vi "功能计算_何 截取位移.vi"(0 "位移数组":dbl[](array[numeric]), 2 "拉压力数组":dbl[](array[numeric])) -> (14 "峰值扭矩":dbl format="%#.2f", 16 "最小扭矩":dbl, 17 "平均扭矩":dbl format="%#.2f", 19 "扭差":dbl format="%#.2f")   [LabVIEW 2013]
panel:
  in  "截取百分比":dbl
  in  "半行程":dbl
  out "第一个子数组":dbl[](array[numeric])
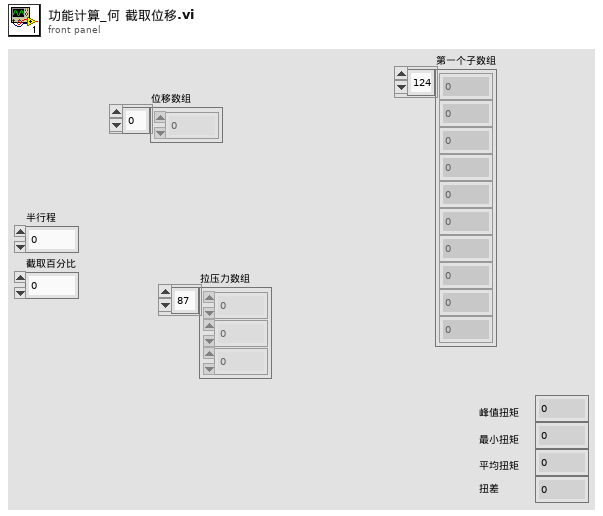
[diagram p1: front panel]
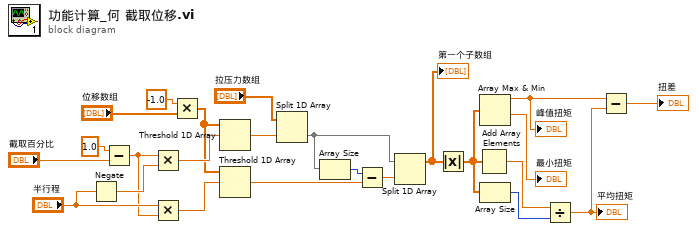
[diagram p0: block diagram]
diagram:
  n1 = Negate(x="半行程") -> (-x=w4:dbl)
  n2 = Subtract(x=1.0, y="截取百分比") -> (x-y=w3:dbl)
  n3 = Multiply(x=w3, y=w4) -> (x*y=w8:dbl)
  n4 = Multiply(x="半行程", y=w3) -> (x*y=w5:dbl)
  n5 = Multiply(x=-1.0, y="位移数组") -> (x*y=w7:dbl[])
  n6 = Threshold 1D Array(2:w8, 3:w7) -> (0:w2:dbl)  [unwired: 1 in]
  n7 = Threshold 1D Array(2:w5, 3:w7) -> (0:w1:dbl)  [unwired: 1 in]
  n8 = Split 1D Array(array="拉压力数组", index=w2) -> (second subarray=w16:dbl[])  [unwired: 1 out]
  n9 = Array Size(array=w16) -> (size(s)=w15:i32)
  n10 = Subtract(x=w15, y=w1) -> (x-y=w14:dbl)
  n11 = Split 1D Array(array=w16, index=w14) -> (first subarray=w20:dbl[])  [unwired: 1 out]
  "第一个子数组" <- w20
  n12 = Absolute Value(x=w20) -> (abs(x)=w22:dbl[])
  n13 = Add Array Elements(numeric array=w22) -> (sum=w23:dbl)
  n14 = Array Max & Min(array=w22) -> (max value=w19:dbl, min value=→"最小扭矩":dbl)  [unwired: 2 out]
  "峰值扭矩" <- w19
  n15 = Array Size(array=w22) -> (size(s)=w21:i32)
  n16 = Divide(x=w23, y=w21) -> (x/y=w18:dbl)
  "平均扭矩" <- w18
  n17 = Subtract(x=w19, y=w18) -> (x-y=→"扭差":dbl)
